vi "Get_card_info_and_handle.vi"(8 "error in (no error)":errorcluster, 11 "Initialize_card in":refnum<class "Initialize_card.lvclass">) -> (0 "error out":errorcluster, 3 "Initialize_card out":refnum<class "Initialize_card.lvclass">)   [LabVIEW 2015, in "Initialize_card.lvclass"]
uses:
  Initialize_card.lvclass
panel:
  out "Sample Bits":i32
  out "Board Count":i32
  out "Channel Count":i32
  out "Trigger Count":i32
  out "System Name":string
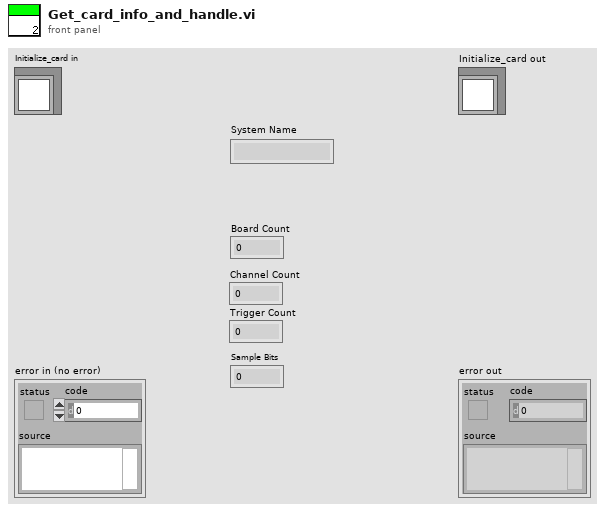
[diagram p1: front panel]
types:
  T1 = cluster{"Handle":u32, "Sample size":u32, "Resolution":i32, "Offset":i32, "Channels":u32, "Boards":u32}
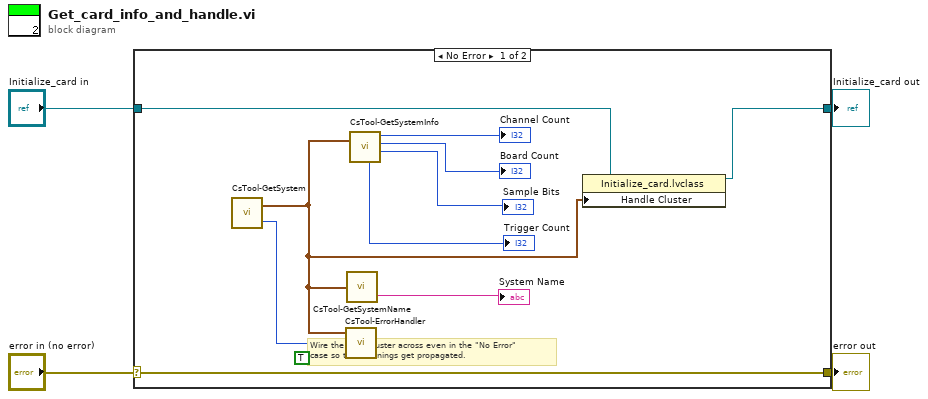
[diagram p0: block diagram]
diagram:
  n1 = case shown="No Error" "error in (no error)" {
    selector: "error in (no error)" -> [w15 w17]
    tunnel: [w15 w17] -> w3
    tunnel: [w6 w16] -> w1
    tunnel: "Initialize_card in" -> [w7 w16]
    frame No Error {
      # "Wire the error cluster across even in the \"No Error\"\ncase so that warnings get propagated."
      n2 = call <userlib>:"CsTool-GetSystem.vi"() -> ("Error Code"=w11:i32, "Handle Cluster"=w5:T1)  [unwired: 4 in]
      n3 = call <userlib>:"CsTool-ErrorHandler.vi"("StopOnError (true)"=TRUE, "Error Code"=w11, "Handle Cluster"=w5) -> ()  [unwired: 1 out]
      n4 = call <userlib>:"CsTool-GetSystemName.vi"("Handle Cluster"=w5) -> ("System Name"=→"System Name":string)  [unwired: 1 out]
      n5 = call <userlib>:"CsTool-GetSystemInfo.vi"("Handle Cluster"=w5) -> ("Number Of Triggers"=→"Trigger Count":u32, "Number Of Channels"=→"Channel Count":u32, "Number Of Boards"=→"Board Count":u32, "Sample Bits"=→"Sample Bits":u32)  [unwired: 3 out]
      n6 = property class="Initialize_card.lvclass"(reference=w7, "Handle Cluster"=w5) -> (reference out=w6:refnum<class "Initialize_card.lvclass">)  [unwired: 1 in, 1 out]
    }
    frame Error {
    }
  }
  "error out" <- w3
  "Initialize_card out" <- w1
